vi "idn_action.vi"(0 "HGF_VISADevice":refnum<class "HGF_VISADevice.lvclass">, 5 "error in (no error)":errorcluster) -> (12 "resourceString":string, 13 "additionalInfo":string, 14 "dup HGF_VISADevice":refnum<class "HGF_VISADevice.lvclass">, 15 "driverRevision":string="unknown", 16 "firmwareRevision":string="unknown", 17 "vendor":string="unknown", 18 "model":string="unknown", 19 "error out":errorcluster)   [LabVIEW 2014, in "HGF_DeviceBaseClasses.lvlib" / "HGF_VISADevice.lvclass"]
doc: "This VI queries the current instrument firmware revision and instrument driver revision.\n\nFor detailed driver information including modification history, refer to the Readme file.\n\n<b>Hint:</b> This is a dynamic dispatch VI to be implemented by child classes."
uses:
  HGF_VISADevice.lvclass
  HGF_DeviceBase/HGF_DeviceBase.lvclass
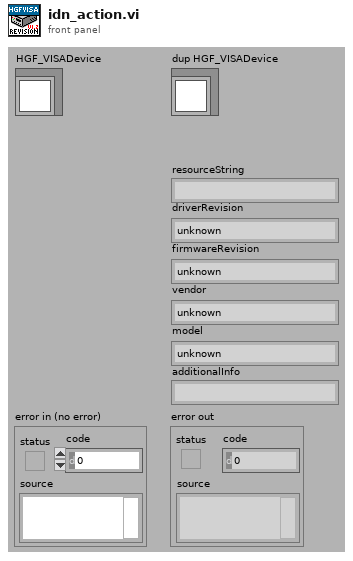
[diagram p1: front panel]
types:
  T1 = cluster{"Baud Rate":u32, "Flow Control":u16, "Parity":u16, "Data Bits":u16, "Stop Bits":u16}
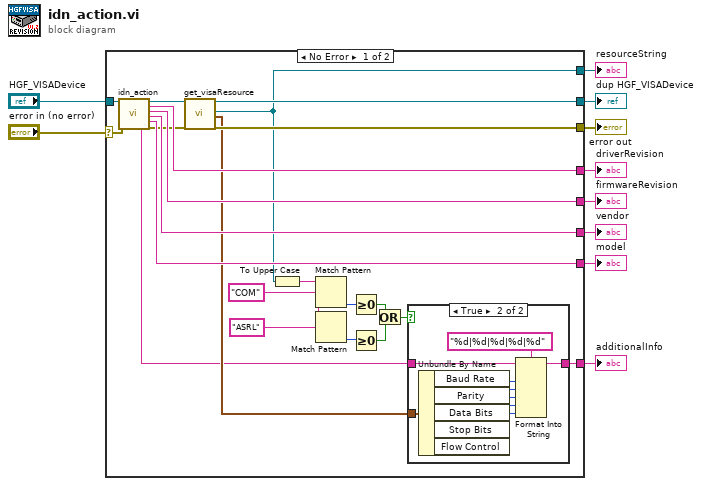
[diagram p0: block diagram]
diagram:
  n1 = case shown="No Error" "error in (no error)" {
    selector: "error in (no error)" -> [w11 w43]
    tunnel: [w32 _] -> w10
    tunnel: [w31 _] -> w9
    tunnel: [w30 _] -> w8
    tunnel: [w29 _] -> w7
    tunnel: "HGF_VISADevice" -> [w28 w44]
    tunnel: [w26 w44] -> w5
    tunnel: [w24 w43] -> w4
    tunnel: [w23 _] -> w3
    tunnel: [w13 _] -> w2
    frame No Error {
      n2 = call-parent "idn_action.vi"("HGF_DeviceBase"=w28, "error in (no error)"=w11) -> ("additionalInfo"=w14:string, "dup HGF_DeviceBase"=w27:refnum<class "HGF_VISADevice.lvclass">, "driverRevision"=w32:string, "firmwareRevision"=w31:string, "vendor"=w30:string, "model"=w29:string, "error out"=w25:errorcluster)  [unwired: 11 out]
      n3 = call "get_visaResource.vi"("HGF_VISADevice"=w27, "error in (no error)"=w25) -> ("dup HGF_VISADevice"=w26:refnum<class "HGF_VISADevice.lvclass">, "VISA Resource Name"=w23:refnum<visa-resource-name>, "Serial Configuration"=w15:T1, "error out"=w24:errorcluster)  [unwired: 14 out]
      n4 = To Upper Case(1:w23) -> (0:w21:string)
      n5 = Match Pattern(string=w21, regular expression="COM") -> (offset past match=w19:i32)  [unwired: 4 out]
      n6 = Match Pattern(string=w21, regular expression="ASRL") -> (offset past match=w18:i32)  [unwired: 4 out]
      n7 = Greater Or Equal To 0?(x=w19) -> (x >= 0?=w17:bool)
      n8 = Greater Or Equal To 0?(x=w18) -> (x >= 0?=w16:bool)
      n9 = Or(x=w17, y=w16) -> (x .or. y?=w12:bool)
      n10 = case shown="True" w12 {
        tunnel: w15 -> [_ w42]
        tunnel: w14 -> [w33 w41]
        tunnel: [w33 w40] -> w13
        frame False {
        }
        frame True {
          n11 = Unbundle By Name(w42) -> ("Baud Rate"=w39:u32, "Parity"=w38:u16, "Data Bits"=w37:u16, "Stop Bits"=w36:u16, "Flow Control"=w35:u16)
          n12 = Format Into String(format string="%d|%d|%d|%d|%d", initial string=w41, w39, w38, w37, w36, w35) -> (resulting string=w40:string)  [unwired: 1 in, 1 out]
        }
      }
    }
    frame Error {
    }
  }
  "error out" <- w4
  "dup HGF_VISADevice" <- w5
  "driverRevision" <- w10
  "firmwareRevision" <- w9
  "vendor" <- w8
  "model" <- w7
  "resourceString" <- w3
  "additionalInfo" <- w2
